vi "SaveSystemDefinitionFile.vi"(8 "error in (no error)":errorcluster, 10 "System Definition File in":path, 11 "System Definition Reference in":refnum<k24>) -> (0 "error out":errorcluster, 3 "System Definition Reference out":refnum<k24>)   [LabVIEW 2015, in "VeriStandTestUtilities.lvlib"]
uses:
  VeriStandTestUtilities.lvlib
  NationalInstruments.VeriStand.SystemDefinitionAPI
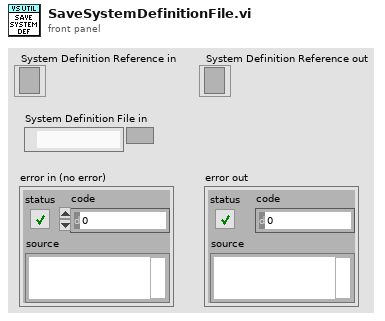
[diagram p1: front panel]
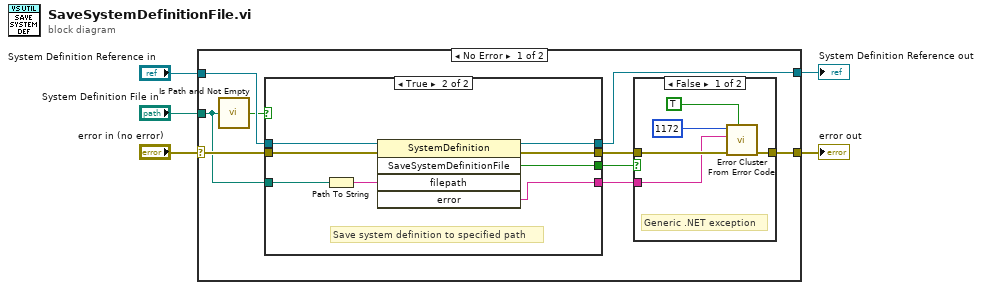
[diagram p0: block diagram]
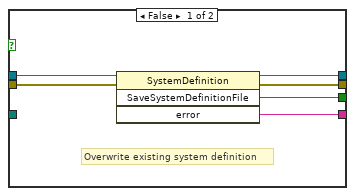
[diagram p2: hidden frame]
diagram:
  n1 = case shown="No Error" "error in (no error)" {
    selector: "error in (no error)" -> [w8 w35]
    tunnel: [w14 w36] -> w5
    tunnel: "System Definition Reference in" -> [w13 w36]
    tunnel: [w9 w35] -> w3
    tunnel: "System Definition File in" -> [w6 _]
    frame No Error {
      n2 = call <vilib>:"Is Path and Not Empty.vi"("path"=w6) -> ("Is Path and Not Empty?"=w7:bool)  [unwired: 4 in]
      n3 = case shown="True" w7 {
        tunnel: [w20 w26] -> w14
        tunnel: w13 -> [w19 w28]
        tunnel: [w18 w24] -> w12
        tunnel: [w17 w25] -> w11
        tunnel: [w16 w21] -> w10
        tunnel: w8 -> [w15 w27]
        tunnel: w6 -> [_ w22]
        frame False {
          # "Overwrite existing system definition"
          n4 = invoke class="SystemDefinition" method="SaveSystemDefinitionFile"(reference=w19, error in=w15) -> (reference out=w20:refnum<k24>, error out=w17:errorcluster, "SaveSystemDefinitionFile"=w18:bool, "error"=w16:string)  [unwired: 2 in]
        }
        frame True {
          # "Save system definition to specified path"
          n5 = Path To String(path=w22) -> (string=w23:string)
          n6 = invoke class="SystemDefinition" method="SaveSystemDefinitionFile"(reference=w28, error in=w27, "filepath"=w23) -> (reference out=w26:refnum<k24>, error out=w25:errorcluster, "SaveSystemDefinitionFile"=w24:bool, "error"=w21:string)  [unwired: 2 in, 1 out]
        }
      }
      n7 = case shown="False" w12 {
        tunnel: [w32 w34] -> w9
        tunnel: w11 -> [w33 w34]
        tunnel: w10 -> [w30 _]
        frame False {
          # "Generic .NET exception"
          n8 = call <vilib>:"Error Cluster From Error Code.vi"("show call chain? (False)"=TRUE, "error in (no error)"=w33, "error message (\"\")"=w30, "error code (0)"=1172) -> ("error out"=w32:errorcluster)  [unwired: 5 in]
        }
        frame True {
        }
      }
    }
    frame Error {
    }
  }
  "System Definition Reference out" <- w5
  "error out" <- w3
